vi "CAPFM-Apply Pause.vi"(0 "Pause Ref":refnum<vi>, 7 "Pause Msg Ref":refnum<vi>, 11 "error in (no error)":errorcluster) -> (15 "error out":errorcluster)   [LabVIEW 2020]
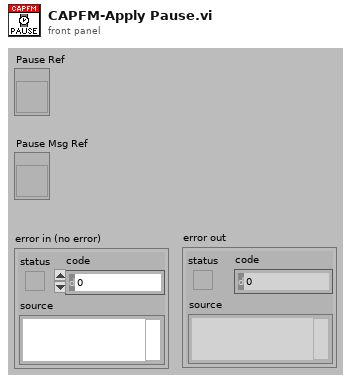
[diagram p1: front panel]
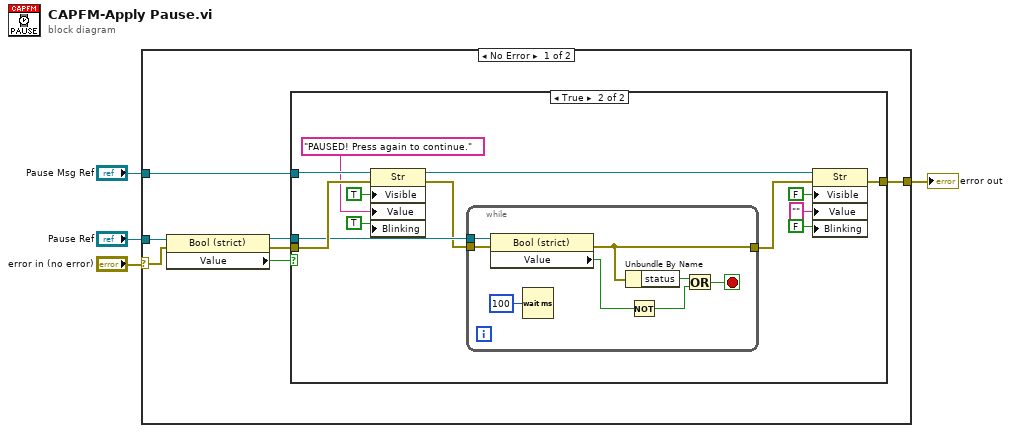
[diagram p0: block diagram]
diagram:
  n1 = case shown="No Error" "error in (no error)" {
    selector: "error in (no error)" -> [w7 w34]
    tunnel: [w5 w34] -> w3
    tunnel: "Pause Ref" -> [w11 _]
    tunnel: "Pause Msg Ref" -> [w8 _]
    frame No Error {
      n2 = property class="Bool (strict)"(reference=w11, error in=w7) -> (reference out=w9:refnum<vi>, error out=w6:errorcluster, "Value"=w10:bool)
      n3 = case shown="True" w10 {
        tunnel: w9 -> [_ w21]
        tunnel: w8 -> [_ w25]
        tunnel: w6 -> [w12 w24]
        tunnel: [w12 w15] -> w5
        frame False {
        }
        frame True {
          n4 = property class="Str"(reference=w25, error in=w24, "Visible"=TRUE, "Value"="PAUSED! Press again to continue.", "Blinking"=TRUE) -> (reference out=w19:refnum<vi>, error out=w20:errorcluster)
          n5 = while {
            tunnel: w21 -> [w33]
            tunnel: w20 -> [w32]
            tunnel: [w26] -> w18
            stop <- w27 stop-if-true
            n6 = property class="Bool (strict)"(reference=w33, error in=w32) -> (error out=w26:errorcluster, "Value"=w30:bool)  [unwired: 1 out]
            n7 = Wait (ms)(milliseconds to wait=u32 100) -> ()  [unwired: 1 out]
            n8 = Unbundle By Name(w26) -> ("status"=w29:bool)
            n9 = Not(x=w30) -> (.not. x?=w28:bool)
            n10 = Or(x=w29, y=w28) -> (x .or. y?=w27:bool)
          }
          n11 = property class="Str"(reference=w19, error in=w18, "Visible"=FALSE, "Value"="", "Blinking"=FALSE) -> (error out=w15:errorcluster)  [unwired: 1 out]
        }
      }
    }
    frame Error {
    }
  }
  "error out" <- w3
